vi "SwerveDrive2.0.vi"(6 "Right Trigger":dbl, 8 "RCW":dbl(slide) scale=-1.0..1.0, 9 "STR":dbl(slide) scale=-1.0..1.0, 10 "FWD":dbl(slide) scale=-1.0..1.0, 11 "Gyro":dbl=-0.03423117662966245) -> ()   [LabVIEW 2023]
uses:
  <vilib>/Rock Robotics/WPI/ThirdParty/ADI/ADIS16470/Typedef/ADIS16470 Data.ctl
  <vilib>/Rock Robotics/WPI/ThirdParty/REV Robotics/REVLib/Typedef/Spark MAX Control Type.ctl
  <vilib>/addons/control/pid/NI_PID_pid.lvlib
  <vilib>/addons/control/pid/pid.llb/PID (DBL).vi
panel:
  in  "Do X Pattern":bool=TRUE
  in  "W4 PID":T1={"proportional gain (Kc)"=0.2, "integral time (Ti, min)"=0.0, "derivative time (Td, min)"=0.0}
  in  "W1 PID":T1={"proportional gain (Kc)"=0.2, "integral time (Ti, min)"=0.0, "derivative time (Td, min)"=0.0}
  in  "W2 PID":T1={"proportional gain (Kc)"=0.2, "integral time (Ti, min)"=0.0, "derivative time (Td, min)"=0.0}
  in  "W3 PID":T1={"proportional gain (Kc)"=0.2, "integral time (Ti, min)"=0.0, "derivative time (Td, min)"=0.0}
  out "ADIS16470 Value":T2
  out "W2 Encoder":dbl
  out "W1 Encoder":dbl
  out "WA 4":dbl=135.0
  out "WA 3":dbl=225.0
  out "WA 2":dbl=315.0
  out "WA 1":dbl=45.0
  out "WS 4":dbl
  out "WS 3":dbl
  out "WS 2":dbl
  out "WS 1":dbl
  out "W4 Encoder":dbl
  out "W3 Encoder":dbl
  # "0.2\n0\n0\nfor all"
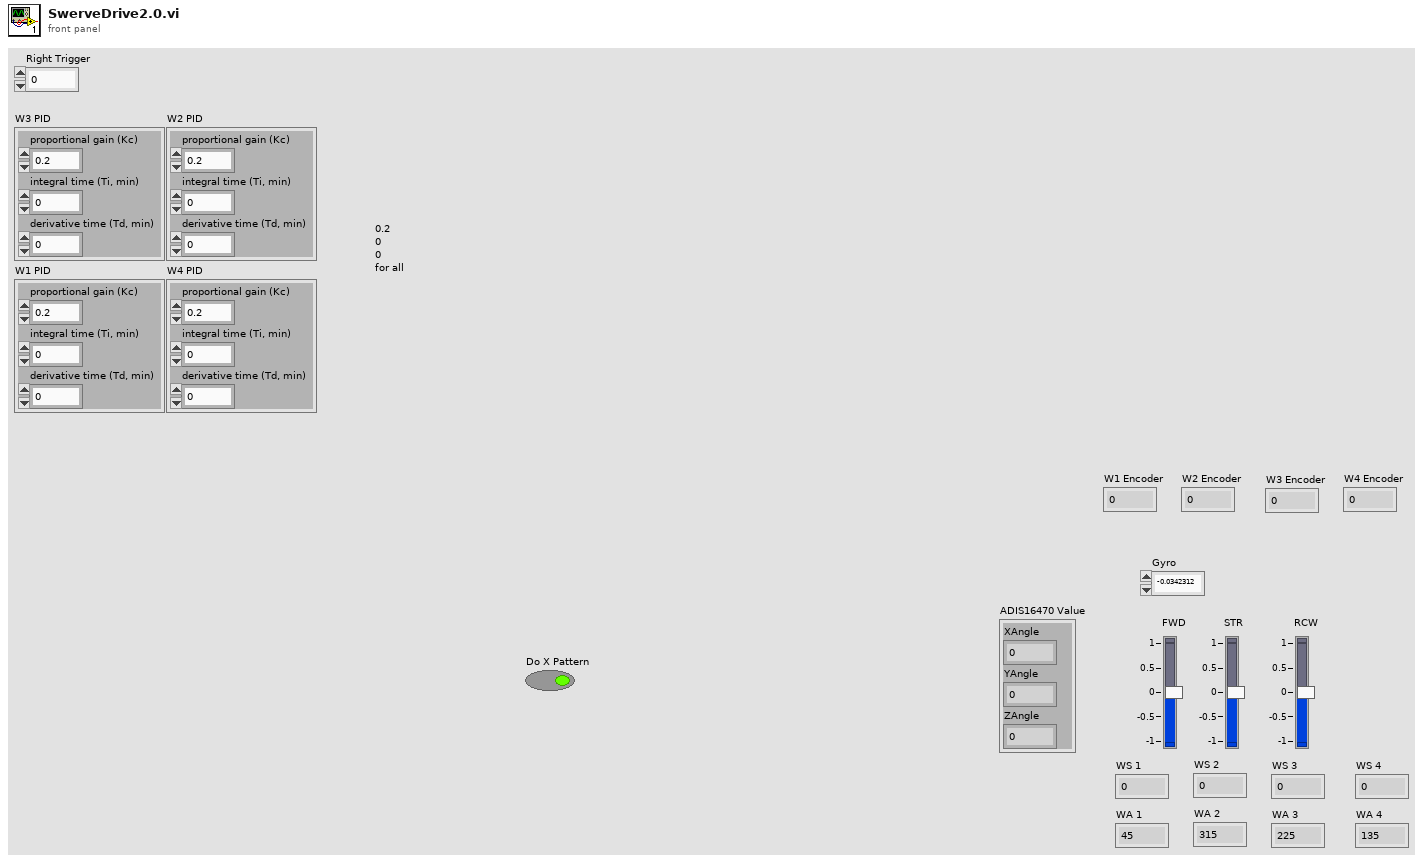
[diagram p1: front panel]
types:
  T1 = cluster{"proportional gain (Kc)":dbl, "integral time (Ti, min)":dbl, "derivative time (Td, min)":dbl}
  T2 = typedef "ADIS16470 Data.ctl" = cluster{"XAngle":dbl, "YAngle":dbl, "ZAngle":dbl}
  T3 = typedef "WPI_JoystickDevRef.ctl" = cluster{"Device":T4}
  T4 = typedef "WPI_JoystickDeviceEnum.ctl" = enum16{"USB 0", "USB 1", "USB 2", "USB 3", "USB 4", "USB 5"}
  T5 = typedef "ADIS16470 Device Reference.ctl" = cluster{"DevStatus":errorcluster, "Hardware Config":T6, "Calibration Complete":refnum<notifier>, "Status Reference":refnum<data-value>, "Data Reference":refnum<data-value>, "Sychronous Process VI":T10, "Cmd FIFO":refnum<k33>, "Source":T11, "Data FIFO":refnum<k33>, "Calibration Time (ms)":u32, "Data Reference":refnum<data-value>}
  T6 = typedef "ADIS16470 Hardware Configuration.ctl" = cluster{"SPI Clock Rate (Hz)":dbl, "IMU SPI Mode (3)":T7, "IMU Reset Pin":T8, "IMU SPI Bus":T9, "IMU Data Ready Pin":T8, "Stall Config":cluster{"Pow2BytesPerRead":u8, "StallTicks":u16, "CsToSclkTicks":u8}}
  T7 = typedef "WPI_SPIMode.ctl" = enum16{"Mode 0 (Clk Idle Low,Sample on Leading)", "Mode 1 (Clk Idle Low,Sample on Trailing)", "Mode 2 (Clk Idle High,Sample on Leading)", "Mode 3 (Clk Idle High,Sample on Trailing)"}
  T8 = typedef "FPGA_DIOChannel.ctl" = enum8{"DIO 0", "DIO 1", "DIO 2", "DIO 3", "DIO 4", "DIO 5", "DIO 6", "DIO 7", "DIO 8", "DIO 9", "DIO MXP 0", "DIO MXP 1", "DIO MXP 2", "DIO MXP 3", "DIO MXP 4", "DIO MXP 5", "DIO MXP 6", "DIO MXP 7", "DIO MXP 8", "DIO MXP 9", "DIO MXP 10", "DIO MXP 11", "DIO MXP 12", "DIO MXP 13", "DIO MXP 14", "DIO MXP 15", "SPI Port CS1", "SPI Port CS2", "SPI Port CS3", "SPI Port MISO", "SPI Port MOSI", "Invalid"}
  T9 = typedef "spi_bus.ctl" = enum16{"SPI On-Board, CS0", "SPI On-Board, CS1", "SPI On-Board, CS2", "SPI On-Board, CS3", "SPI MXP", "Invalid"}
  T10 = typedef "ADIS16470 Process.ctl" = refnum<vi>
  T11 = typedef "FPGA_CounterEncoderSourceConvertionLVSourceType.ctl" = cluster{"DevStatus":errorcluster, "AnalogTriggerMode?":bool, "DigitalMode":cluster{"DIO Channel":T12}, "AnalogTriggerMode":cluster{"AnalogTriggerIndex":T13, "OutputType":T14}}
  T12 = typedef "FPGA_DIODigitalSourceChannel.ctl" = enum8{"DIO 0", "DIO 1", "DIO 2", "DIO 3", "DIO 4", "DIO 5", "DIO 6", "DIO 7", "DIO 8", "DIO 9", "DIO MXP 0", "DIO MXP 1", "DIO MXP 2", "DIO MXP 3", "DIO MXP 4", "DIO MXP 5", "DIO MXP 6", "DIO MXP 7", "DIO MXP 8", "DIO MXP 9", "DIO MXP 10", "DIO MXP 11", "DIO MXP 12", "DIO MXP 13", "DIO MXP 14", "DIO MXP 15", "SPI Port CS1", "SPI Port CS2", "SPI Port CS3", "SPI Port MISO", "SPI Port MOSI", "Disabled"}
  T13 = typedef "FPGA_AnalogTriggerIndex.ctl" = enum8{"Trig 0", "Trig 1", "Trig 2", "Trig 3", "Trig 4", "Trig 5", "Trig 6", "Trig 7", "Invalid"}
  T14 = typedef "FPGA_AnalogTriggerOutType.ctl" = enum16{"InWindow", "TriggerState", "Rising", "Falling"}
  T15 = typedef "WPI_MotorControlDeviceRef.ctl" = cluster{"DeviceStatus":errorcluster, "Type":T16, "PWM":cluster{"PWM Channel":T17, "DeadBand":T18}, "CAN":cluster{"Device Number":u8, "SetOutput VI Ref":variant, "GetOutput VI Ref":variant, "Enable VI Ref":variant, "Disable VI Ref":variant, "Data":variant}, "Invert":bool, "DIO PWM":cluster{"PWM \"Enable\" Channel":T17, "DIOChannel":T8, "PWM Rate":dbl}}
  T16 = typedef "WPI_MotorControlType.ctl" = enum16{"PWM", "CAN", "DIO PWM"}
  T17 = typedef "FPGA_DIOPWMChannel.ctl" = enum8{"PWM 0", "PWM 1", "PWM 2", "PWM 3", "PWM 4", "PWM 5", "PWM 6", "PWM 7", "PWM 8", "PWM 9", "PWM MXP 0", "PWM MXP 1", "PWM MXP 2", "PWM MXP 3", "PWM MXP 4", "PWM MXP 5", "PWM MXP 6", "PWM MXP 7", "PWM MXP 8", "PWM MXP 9", "Invalid"}
  T18 = typedef "WPI_PWMDeadband.ctl" = cluster{"Name":string, "maxPositivePwm":i32, "minPositivePwm":i32, "centerPwm":i32, "maxNegativePwm":i32, "minNegativePwm":i32, "angularRange":u16}
  T19 = typedef "Spark MAX Control Type.ctl" = enum16{"Percent VBus", "Voltage", "Velocity", "Position", "Smart Motion", "Current", "Smart Velocity"}
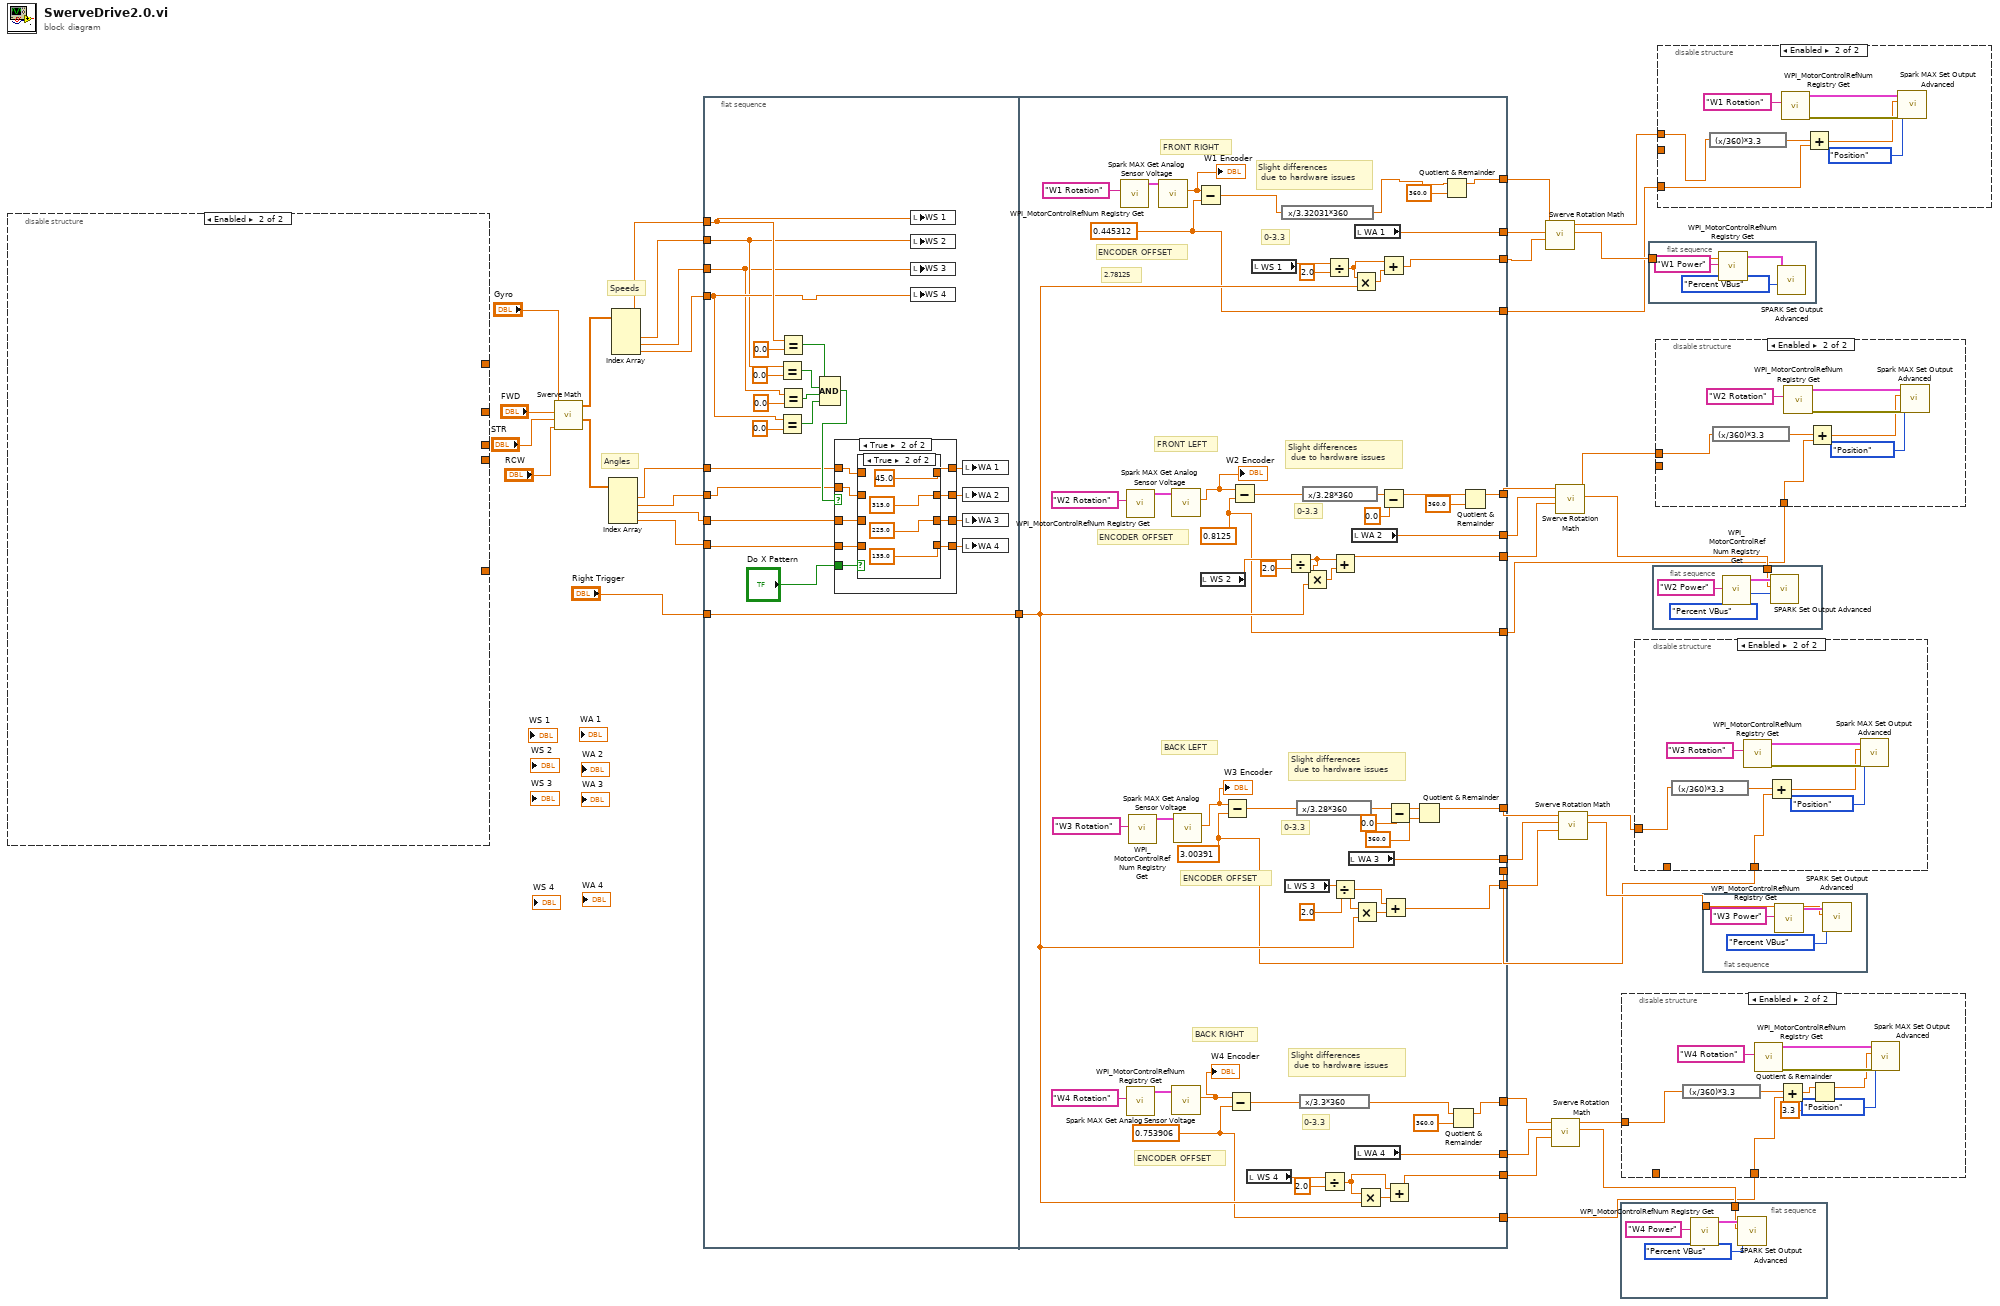
[diagram p0: block diagram]
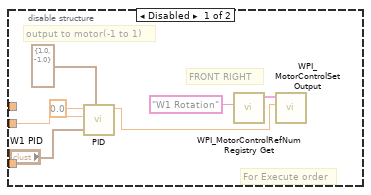
[diagram p2: hidden frame]
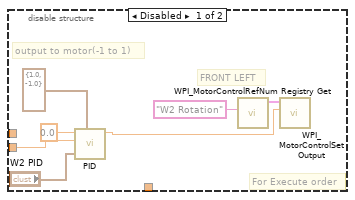
[diagram p3: hidden frame]
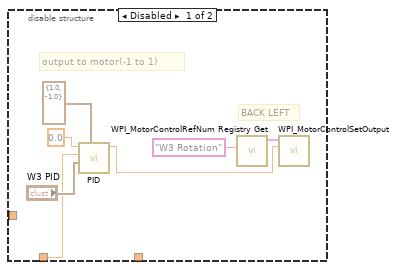
[diagram p4: hidden frame]
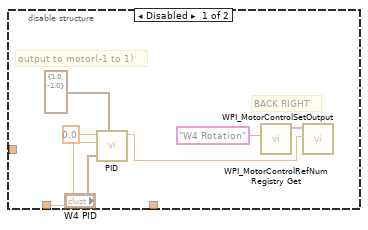
[diagram p5: hidden frame]
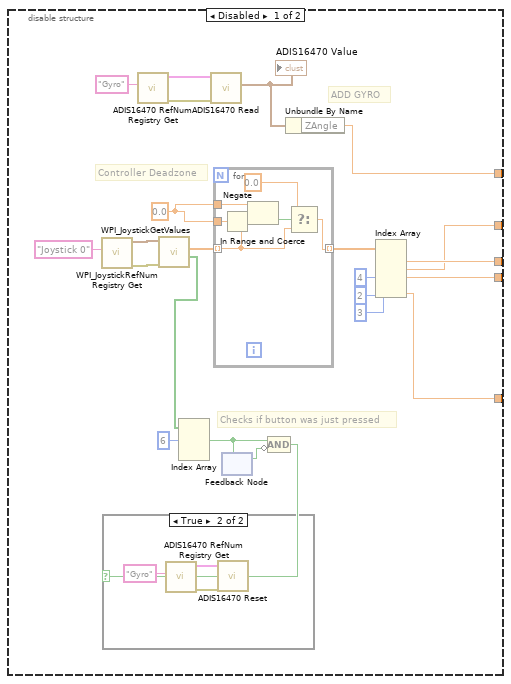
[diagram p6: hidden frame]
diagram:
  # "Angles"
  # "Speeds"
  n1 = disable-structure shown="Enabled" {
    disable-tunnel: [w60 _] -> _
    disable-tunnel: [w59 _] -> _
    disable-tunnel: [w58 _] -> _
    disable-tunnel: [w47 _] -> _
    disable-tunnel: [w44 _] -> _
    frame Disabled {
      w53 = 0.0 ("upper limit")
      # "Checks if button was just pressed"
      # "Controller Deadzone"
      # "ADD GYRO"
      n2 = call <vilib>:"WPI_JoystickRefNum Registry Get.vi"("refnum name"="Joystick 0") -> ("error out"=w63:errorcluster, "JoystickDevRef"=w62:T3)  [unwired: 9 in]
      n3 = call <vilib>:"ADIS16470 RefNum Registry Get.vi"("refnum name"="Gyro") -> ("error out"=w43:errorcluster, "ADIS16470DevRef out"=w41:T5)  [unwired: 9 in]
      n4 = call <vilib>:"WPI_JoystickGetValues.vi"("error in (no error)"=w63, "JoystickDevRef"=w62) -> ("Buttons"=w52:bool[], "Axes"=w55:dbl[])  [unwired: 5 in, 3 out]
      n5 = Index Array(array=w52, index #1=6 ("index")) -> (element #1=w50:bool)  [unwired: 2 in, 2 out]
      n6 = call <vilib>:"ADIS16470 Read.vi"("error in (no error)"=w43, "ADIS16470DevRef"=w41) -> ("ADIS16470 Value"=w56:T2)  [unwired: 6 in, 3 out]
      "ADIS16470 Value" <- w56
      n7 = for {
        tunnel: w55 -> [w68] mode=indexing
        tunnel: [w67] -> w54 mode=indexing
        tunnel: w53 -> [w73]
        tunnel: w53 -> [w72]
        n8 = Negate(x=w72) -> (-x=w71:dbl)
        n9 = In Range and Coerce(upper limit=w73, x=w68, lower limit=w71) -> (In Range?=w70:bool)  [unwired: 1 out]
        n10 = Select(t=0.0, s=w70, f=w68) -> (s? t:f=w67:dbl)
      }
      n11 = feedback #1() -> (w49:bool)  [unwired: 1 in]
      n12 = feedback-in #1(w50) -> ()
      n13 = Compound Arithmetic op=AND(w50, invert w49) -> (w48:bool)
      n14 = case shown="True" w48 {
        frame False {
        }
        frame True {
          n15 = call <vilib>:"ADIS16470 RefNum Registry Get.vi"("refnum name"="Gyro") -> ("error out"=w65:errorcluster, "ADIS16470DevRef out"=w64:T5)  [unwired: 9 in]
          n16 = call <vilib>:"ADIS16470 Reset.vi"("error in (no error)"=w65, "ADIS16470DevRef"=w64) -> ()  [unwired: 8 in, 2 out]
        }
      }
      n17 = Unbundle By Name(w56) -> ("ZAngle"=w47:dbl)
      n18 = Index Array(array=w54, index #3=4 ("index"), index #4=2 ("index"), index #5=3 ("index")) -> (element #1=w60:dbl, element #2=w58:dbl, element #3=w59:dbl, element #5=w44:dbl)  [unwired: 2 in, 1 out]
    }
    frame Enabled {
    }
  }
  n19 = call "Swerve Math.vi"("Gyro"="Gyro", "FWD"="FWD", "STR"="STR", "RCW"="RCW") -> ("Wheel Speeds"=w40:dbl[], "Wheel Angles"=w39:dbl[])  [unwired: 5 in]
  n20 = Index Array(array=w39) -> (element #1=w32:dbl, element #2=w33:dbl, element #3=w34:dbl, element #4=w35:dbl)  [unwired: 4 in]
  n21 = Index Array(array=w40) -> (element #1=w30:dbl, element #2=w28:dbl, element #3=w29:dbl, element #4=w31:dbl)  [unwired: 4 in]
  n22 = flat-sequence {
    tunnel: w35 -> [w77]
    tunnel: w34 -> [w81]
    tunnel: w33 -> [w83]
    tunnel: w32 -> [w85]
    tunnel: w31 -> [w76]
    tunnel: w29 -> [w74]
    tunnel: w30 -> [w87]
    tunnel: w28 -> [w75]
    tunnel: "Right Trigger" -> [w96]
    tunnel: [w96] -> w27
    tunnel: [w178] -> w23
    tunnel: [w177] -> w19
    tunnel: [w131] -> w15
    tunnel: [w176] -> w10
    tunnel: [w132] -> w14
    tunnel: [w140] -> w20
    tunnel: [w138] -> w6
    tunnel: [w155] -> w22
    tunnel: [w159] -> w18
    tunnel: [w151] -> w13
    tunnel: [w149] -> w9
    tunnel: w27 -> [w147]
    tunnel: [w135] -> w11
    tunnel: [w121] -> w4
    tunnel: [w120] -> w3
    tunnel: [w119] -> w2
    tunnel: [w118] -> w1
    frame #0 {
      n23 = Equal?(x=w75, y=0.0) -> (x = y?=w92:bool)
      n24 = Equal?(x=w76, y=0.0) -> (x = y?=w88:bool)
      n25 = Equal?(x=w87, y=0.0) -> (x = y?=w95:bool)
      n26 = Equal?(x=w74, y=0.0) -> (x = y?=w89:bool)
      n27 = Compound Arithmetic op=AND(w95, w92, w89, w88) -> (w86:bool)
      n28 = case shown="True" w86 {
        tunnel: w85 -> [w100 w104]
        tunnel: [w100 w109] -> w84
        tunnel: w83 -> [w99 w103]
        tunnel: [w99 w108] -> w82
        tunnel: w81 -> [w98 w102]
        tunnel: [w98 w107] -> w80
        tunnel: w77 -> [w97 w101]
        tunnel: [w97 w106] -> w79
        tunnel: "Do X Pattern" -> [_ w105]
        frame False {
        }
        frame True {
          n29 = case shown="True" w105 {
            tunnel: [w113 45.0] -> w109
            tunnel: [w112 315.0] -> w108
            tunnel: [w111 225.0] -> w107
            tunnel: [w110 135.0] -> w106
            tunnel: w104 -> [w113 _]
            tunnel: w103 -> [w112 _]
            tunnel: w102 -> [w111 _]
            tunnel: w101 -> [w110 _]
            frame False {
            }
            frame True {
            }
          }
        }
      }
      n30 = local write "WS 1"(w87) -> ()
      n31 = local write "WS 2"(w75) -> ()
      n32 = local write "WS 3"(w74) -> ()
      n33 = local write "WS 4"(w76) -> ()
      n34 = local write "WA 1"(w84) -> ()
      n35 = local write "WA 2"(w82) -> ()
      n36 = local write "WA 3"(w80) -> ()
      n37 = local write "WA 4"(w79) -> ()
    }
    frame #1 {
      w118 = 0.753906 ("x")
      w119 = 3.00391 ("y")
      w120 = 0.8125 ("y")
      w121 = 0.445312 ("y")
      # "2.78125"
      # "Slight differences\n due to hardware issues"
      # "Slight differences\n due to hardware issues"
      # "Slight differences\n due to hardware issues"
      # "Slight differences\n due to hardware issues"
      # "BACK RIGHT"
      # "BACK LEFT"
      # "FRONT LEFT"
      # "FRONT RIGHT"
      # "ENCODER OFFSET"
      # "ENCODER OFFSET"
      # "ENCODER OFFSET"
      # "ENCODER OFFSET"
      # "0-3.3"
      # "0-3.3"
      # "0-3.3"
      # "0-3.3"
      n38 = call <vilib>:"WPI_MotorControlRefNum Registry Get.vi"("refnum name"="W1 Rotation") -> ("MotorControlDevRef"=w175:T15)  [unwired: 9 in, 1 out]
      n39 = call <vilib>:"WPI_MotorControlRefNum Registry Get.vi"("refnum name"="W2 Rotation") -> ("MotorControlDevRef"=w164:T15)  [unwired: 9 in, 1 out]
      n40 = call <vilib>:"WPI_MotorControlRefNum Registry Get.vi"("refnum name"="W4 Rotation") -> ("MotorControlDevRef"=w170:T15)  [unwired: 9 in, 1 out]
      n41 = call <vilib>:"WPI_MotorControlRefNum Registry Get.vi"("refnum name"="W3 Rotation") -> ("MotorControlDevRef"=w172:T15)  [unwired: 9 in, 1 out]
      n42 = call <vilib>:"Spark MAX Get Analog Sensor Voltage.vi"("MotorControlDevRef in"=w175) -> ("Analog Sensor Voltage"=w127:dbl)  [unwired: 7 in, 3 out]
      "W1 Encoder" <- w127
      n43 = call <vilib>:"Spark MAX Get Analog Sensor Voltage.vi"("MotorControlDevRef in"=w164) -> ("Analog Sensor Voltage"=w129:dbl)  [unwired: 7 in, 3 out]
      "W2 Encoder" <- w129
      n44 = call <vilib>:"Spark MAX Get Analog Sensor Voltage.vi"("MotorControlDevRef in"=w170) -> ("Analog Sensor Voltage"=w123:dbl)  [unwired: 7 in, 3 out]
      "W4 Encoder" <- w123
      n45 = call <vilib>:"Spark MAX Get Analog Sensor Voltage.vi"("MotorControlDevRef in"=w172) -> ("Analog Sensor Voltage"=w125:dbl)  [unwired: 7 in, 3 out]
      "W3 Encoder" <- w125
      n46 = Subtract(x=w127, y=w121) -> (x-y=w126:dbl)
      n47 = local read "WS 2"() -> (w167:dbl)
      n48 = Subtract(x=w125, y=w119) -> (x-y=w124:dbl)
      n49 = Subtract(x=w123, y=w118) -> (x-y=w122:dbl)
      n50 = Subtract(x=w129, y=w120) -> (x-y=w128:dbl)
      n51 = local read "WS 4"() -> (w165:dbl)
      n52 = local read "WS 1"() -> (w168:dbl)
      n53 = expression code="x/3.32031*360"(w126) -> (w130:dbl)
      n54 = local read "WS 3"() -> (w166:dbl)
      n55 = Divide(x=w167, y=2.0) -> (x/y=w157:dbl)
      n56 = expression code="x/3.28*360"(w124) -> (w146:dbl)
      n57 = expression code="x/3.3*360"(w122) -> (w136:dbl)
      n58 = expression code="x/3.28*360"(w128) -> (w142:dbl)
      n59 = Multiply(x=w157, y=w147) -> (x*y=w158:dbl)
      n60 = Divide(x=w165, y=2.0) -> (x/y=w148:dbl)
      n61 = Divide(x=w168, y=2.0) -> (x/y=w154:dbl)
      n62 = Add(x=w157, y=w158) -> (x+y=w159:dbl)
      n63 = Divide(x=w166, y=2.0) -> (x/y=w152:dbl)
      n64 = local read "WA 3"() -> (w131:dbl)
      n65 = Multiply(x=w154, y=w147) -> (x*y=w156:dbl)
      n66 = local read "WA 2"() -> (w177:dbl)
      n67 = Multiply(x=w152, y=w147) -> (x*y=w153:dbl)
      n68 = local read "WA 1"() -> (w178:dbl)
      n69 = local read "WA 4"() -> (w176:dbl)
      n70 = Multiply(x=w148, y=w147) -> (x*y=w150:dbl)
      n71 = Add(x=w154, y=w156) -> (x+y=w155:dbl)
      n72 = Subtract(x=w142, y=0.0) -> (x-y=w134:dbl)
      n73 = Add(x=w152, y=w153) -> (x+y=w151:dbl)
      n74 = Add(x=w148, y=w150) -> (x+y=w149:dbl)
      n75 = Subtract(x=w146, y=0.0) -> (x-y=w145:dbl)
      n76 = Quotient & Remainder(x=w145, y=360.0) -> (x-y*floor(x/y)=w132:dbl)  [unwired: 1 out]
      n77 = Quotient & Remainder(x=w130, y=360.0) -> (x-y*floor(x/y)=w138:dbl)  [unwired: 1 out]
      n78 = Quotient & Remainder(x=w136, y=360.0) -> (x-y*floor(x/y)=w135:dbl)  [unwired: 1 out]
      n79 = Quotient & Remainder(x=w134, y=360.0) -> (x-y*floor(x/y)=w140:dbl)  [unwired: 1 out]
    }
  }
  n80 = call "Swerve Rotation Math.vi"("Wheel Speed"=w22, "Wheel Angle"=w23, "Encoder"=w6) -> ("Wheel Speed"=w24:dbl, "Goal"=w25:dbl)  [unwired: 7 in]
  n81 = call "Swerve Rotation Math.vi"("Wheel Speed"=w9, "Wheel Angle"=w10, "Encoder"=w11) -> ("Wheel Speed"=w8:dbl, "Goal"=w7:dbl)  [unwired: 7 in]
  n82 = call "Swerve Rotation Math.vi"("Wheel Speed"=w18, "Wheel Angle"=w19, "Encoder"=w20) -> ("Wheel Speed"=w17:dbl, "Goal"=w21:dbl)  [unwired: 7 in]
  n83 = call "Swerve Rotation Math.vi"("Wheel Speed"=w13, "Wheel Angle"=w15, "Encoder"=w14) -> ("Wheel Speed"=w12:dbl, "Goal"=w16:dbl)  [unwired: 7 in]
  n84 = flat-sequence {
    tunnel: w8 -> [w180]
    frame #0 {
      n85 = call <vilib>:"WPI_MotorControlRefNum Registry Get.vi"("refnum name"="W4 Power") -> ("MotorControlDevRef"=w181:T15)  [unwired: 9 in, 1 out]
      n86 = call <vilib>:"SPARK Set Output Advanced.vi"("Control Mode"=Spark_MAX_Control_Type."Percent VBus", "Setpoint"=w180, "MotorControlDevRef"=w181) -> ()  [unwired: 7 in, 2 out]
    }
  }
  n87 = disable-structure shown="Enabled" {
    disable-tunnel: _ -> [w190 _]
    disable-tunnel: w7 -> [_ w195]
    disable-tunnel: w1 -> [_ w191]
    frame Disabled {
      # "output to motor(-1 to 1)"
      # "BACK RIGHT"
      n88 = call-poly <vilib>:"PID.vi"("output range"=cluster{"output high":dbl, "output low":dbl} {"output high"=1.0, "output low"=-1.0}, "PID gains"="W4 PID", "process variable"=w190, "setpoint"=0.0) -> ("output"=w188:dbl)  [unwired: 6 in, 1 out]
      n89 = call <vilib>:"WPI_MotorControlRefNum Registry Get.vi"("refnum name"="W4 Rotation") -> ("MotorControlDevRef"=w189:T15)  [unwired: 9 in, 1 out]
      n90 = call <vilib>:"WPI_MotorControlSetOutput.vi"("Output"=w188, "MotorControlDevRef"=w189) -> ("Motor Output"=w186:dbl)  [unwired: 7 in, 2 out]
    }
    frame Enabled {
      n91 = expression code="(x/360)*3.3"(w195) -> (w196:dbl)
      n92 = call <vilib>:"WPI_MotorControlRefNum Registry Get.vi"("refnum name"="W4 Rotation") -> ("error out"=w197:errorcluster, "MotorControlDevRef"=w198:T15)  [unwired: 9 in]
      n93 = Add(x=w196, y=w191) -> (x+y=w194:dbl)
      n94 = Quotient & Remainder(x=w194, y=3.3) -> (x-y*floor(x/y)=w192:dbl)  [unwired: 1 out]
      n95 = call <vilib>:"Spark MAX Set Output Advanced.vi"("error in (no error)"=w197, "Control Mode"=Spark_MAX_Control_Type."Position", "Setpoint"=w192, "MotorControlDevRef"=w198) -> ()  [unwired: 6 in, 2 out]
    }
  }
  n96 = disable-structure shown="Enabled" {
    disable-tunnel: _ -> [w204 _]
    disable-tunnel: w16 -> [_ w209]
    disable-tunnel: w2 -> [_ w208]
    frame Disabled {
      # "BACK LEFT"
      # "output to motor(-1 to 1)"
      n97 = call-poly <vilib>:"PID.vi"("output range"=cluster{"output high":dbl, "output low":dbl} {"output high"=1.0, "output low"=-1.0}, "PID gains"="W3 PID", "process variable"=w204, "setpoint"=0.0) -> ("output"=w202:dbl)  [unwired: 6 in, 1 out]
      n98 = call <vilib>:"WPI_MotorControlRefNum Registry Get.vi"("refnum name"="W3 Rotation") -> ("MotorControlDevRef"=w203:T15)  [unwired: 9 in, 1 out]
      n99 = call <vilib>:"WPI_MotorControlSetOutput.vi"("Output"=w202, "MotorControlDevRef"=w203) -> ()  [unwired: 7 in, 3 out]
    }
    frame Enabled {
      n100 = expression code="(x/360)*3.3"(w209) -> (w211:dbl)
      n101 = call <vilib>:"WPI_MotorControlRefNum Registry Get.vi"("refnum name"="W3 Rotation") -> ("error out"=w212:errorcluster, "MotorControlDevRef"=w213:T15)  [unwired: 9 in]
      n102 = Add(x=w211, y=w208) -> (x+y=w210:dbl)
      n103 = call <vilib>:"Spark MAX Set Output Advanced.vi"("error in (no error)"=w212, "Control Mode"=Spark_MAX_Control_Type."Position", "Setpoint"=w210, "MotorControlDevRef"=w213) -> ()  [unwired: 6 in, 2 out]
    }
  }
  n104 = flat-sequence {
    tunnel: w24 -> [w217]
    frame #0 {
      n105 = call <vilib>:"WPI_MotorControlRefNum Registry Get.vi"("refnum name"="W1 Power") -> ("MotorControlDevRef"=w218:T15)  [unwired: 9 in, 1 out]
      n106 = call <vilib>:"SPARK Set Output Advanced.vi"("Control Mode"=Spark_MAX_Control_Type."Percent VBus", "Setpoint"=w217, "MotorControlDevRef"=w218) -> ()  [unwired: 7 in, 2 out]
    }
  }
  n107 = flat-sequence {
    tunnel: w17 -> [w221]
    frame #0 {
      n108 = call <vilib>:"WPI_MotorControlRefNum Registry Get.vi"("refnum name"="W2 Power") -> ("MotorControlDevRef"=w222:T15)  [unwired: 9 in, 1 out]
      n109 = call <vilib>:"SPARK Set Output Advanced.vi"("Control Mode"=Spark_MAX_Control_Type."Percent VBus", "Setpoint"=w221, "MotorControlDevRef"=w222) -> ()  [unwired: 7 in, 2 out]
    }
  }
  n110 = disable-structure shown="Enabled" {
    disable-tunnel: _ -> [w228 _]
    disable-tunnel: w21 -> [_ w233]
    disable-tunnel: w3 -> [_ w232]
    frame Disabled {
      # "FRONT LEFT"
      # "output to motor(-1 to 1)"
      # "For Execute order"
      n111 = call-poly <vilib>:"PID.vi"("output range"=cluster{"output high":dbl, "output low":dbl} {"output high"=1.0, "output low"=-1.0}, "PID gains"="W2 PID", "process variable"=w228, "setpoint"=0.0) -> ("output"=w226:dbl)  [unwired: 6 in, 1 out]
      n112 = call <vilib>:"WPI_MotorControlRefNum Registry Get.vi"("refnum name"="W2 Rotation") -> ("MotorControlDevRef"=w227:T15)  [unwired: 9 in, 1 out]
      n113 = call <vilib>:"WPI_MotorControlSetOutput.vi"("Output"=w226, "MotorControlDevRef"=w227) -> ("Motor Output"=w224:dbl)  [unwired: 7 in, 2 out]
    }
    frame Enabled {
      n114 = expression code="(x/360)*3.3"(w233) -> (w235:dbl)
      n115 = call <vilib>:"WPI_MotorControlRefNum Registry Get.vi"("refnum name"="W2 Rotation") -> ("error out"=w236:errorcluster, "MotorControlDevRef"=w237:T15)  [unwired: 9 in]
      n116 = Add(x=w235, y=w232) -> (x+y=w234:dbl)
      n117 = call <vilib>:"Spark MAX Set Output Advanced.vi"("error in (no error)"=w236, "Control Mode"=Spark_MAX_Control_Type."Position", "Setpoint"=w234, "MotorControlDevRef"=w237) -> ()  [unwired: 6 in, 2 out]
    }
  }
  n118 = disable-structure shown="Enabled" {
    disable-tunnel: _ -> [w244 _]
    disable-tunnel: w25 -> [_ w249]
    disable-tunnel: w4 -> [_ w248]
    frame Disabled {
      # "FRONT RIGHT"
      # "output to motor(-1 to 1)"
      # "For Execute order"
      n119 = call-poly <vilib>:"PID.vi"("output range"=cluster{"output high":dbl, "output low":dbl} {"output high"=1.0, "output low"=-1.0}, "PID gains"="W1 PID", "process variable"=w244, "setpoint"=0.0) -> ("output"=w242:dbl)  [unwired: 6 in, 1 out]
      n120 = call <vilib>:"WPI_MotorControlRefNum Registry Get.vi"("refnum name"="W1 Rotation") -> ("MotorControlDevRef"=w243:T15)  [unwired: 9 in, 1 out]
      n121 = call <vilib>:"WPI_MotorControlSetOutput.vi"("Output"=w242, "MotorControlDevRef"=w243) -> ("Motor Output"=w240:dbl)  [unwired: 7 in, 2 out]
    }
    frame Enabled {
      n122 = expression code="(x/360)*3.3"(w249) -> (w251:dbl)
      n123 = call <vilib>:"WPI_MotorControlRefNum Registry Get.vi"("refnum name"="W1 Rotation") -> ("error out"=w252:errorcluster, "MotorControlDevRef"=w253:T15)  [unwired: 9 in]
      n124 = Add(x=w251, y=w248) -> (x+y=w250:dbl)
      n125 = call <vilib>:"Spark MAX Set Output Advanced.vi"("error in (no error)"=w252, "Control Mode"=Spark_MAX_Control_Type."Position", "Setpoint"=w250, "MotorControlDevRef"=w253) -> ()  [unwired: 6 in, 2 out]
    }
  }
  n126 = flat-sequence {
    tunnel: w12 -> [w257]
    frame #0 {
      n127 = call <vilib>:"WPI_MotorControlRefNum Registry Get.vi"("refnum name"="W3 Power") -> ("MotorControlDevRef"=w258:T15)  [unwired: 9 in, 1 out]
      n128 = call <vilib>:"SPARK Set Output Advanced.vi"("Control Mode"=Spark_MAX_Control_Type."Percent VBus", "Setpoint"=w257, "MotorControlDevRef"=w258) -> ()  [unwired: 7 in, 2 out]
    }
  }
